vi "PI_GCS2_Sample_Application_With_Analog.vi"() -> ()   [LabVIEW 2020]
doc: "This VI demonstrates the use of digital (e.g. RS-232) communication and analog interfacing in parallel for a PI GCS2 device which can be operated in analog mode. In this example the PI GCS2 device is connected through COM port 1 with baudrate 115200. The VI first initializes the device via the selected digital interface by running PI_GCS2_Configuration_Setup.vi. It then switches to analog control using SwitchToAnalogOrDigital.vi and initializes the analog interface by running Analog_Configuration_Setup.vi. After these initialization steps, it moves one axis relative to its current position by outputting a voltage by the DAC card used, waits 10 ms and queries for the position of this axis. Finally, it switches back to digital control and closes both the analog and the digital connection to the device. \nThe diagram shows how to combine the driver VIs for these tasks. \nWarning: Before running this VI, modify the interface settings to reflect your configuration. The predefined settings provided with the VI probably do not match your system."
uses:
  Low Level/Communication.llb/Interface Settings.ctl
panel:
  out "Running 2":bool caption="Analog_Configuration_Setup.vi is running"
  in  "stop":bool
  in  "error in":errorcluster
  out "Running":bool caption="PI_GCS2_Configuration_Setup.vi is running"
  out "error out":errorcluster
  out "Position":dbl[](array[numeric]) format="%.6f"
  out "Conn. Axis":string[](array[string])
  out "GCS2 Identification":string
  # "This This VI demonstrates the use of digital (e.g. RS-232) communication and analog interfacing in parallel for a PI CGS2 devie that can be operated in analog mode.  The diagram shows how to combine the driver VIs for these tasks.\n\nWarning: Before running this VI, modify the interface settings on the block diagram to reflect your configuration. The predefined \n                 settings provided with the VI probably do not match your system.\n                 Both the PI GCS2 LabVIEW driver set and the GCS Analog LabVIEW driver set must be installed, otherwise the VI will not\n                 be executable."
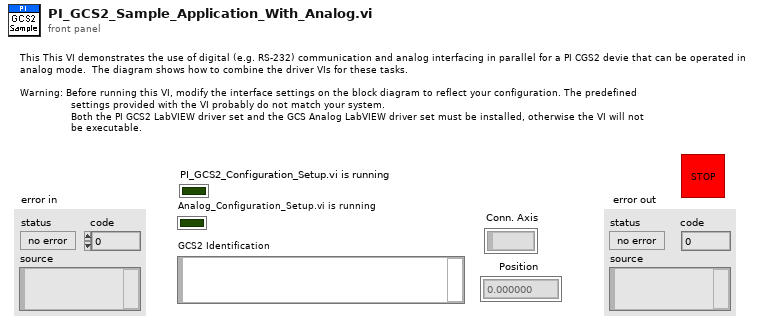
[diagram p1: front panel]
types:
  T1 = typedef "Interface Settings.ctl" = cluster{"Interface":u16, "Timeout":u32, "RS232 settings":cluster{"Portnumber":u8, "Baudrate":u16}, "TCP/IP settings":cluster{"Host address/name":string, "Port":i32, "Board":i32, "TCP/IP Search?":bool}, "USB settings":cluster{"S/N":string, "USB Search?":bool}, "DaisyChain settings":cluster{"Register DC":bool, "DaisyChain Search?":bool, "Device ID":i32}, "DLL for Device":u16}
  T2 = enum16{"Do not reference", "Reference switch", "Negative limit switch", "Positive limit switch"}[]
  T3 = cluster{"Conn. Axes":string[], "AI channels":tag[], "AO channels":tag[], "Lower voltage limit (V)":dbl, "Upper voltage limit (V)":dbl, "AI Sample Rate":dbl, "AI Samples/Channel":i32}
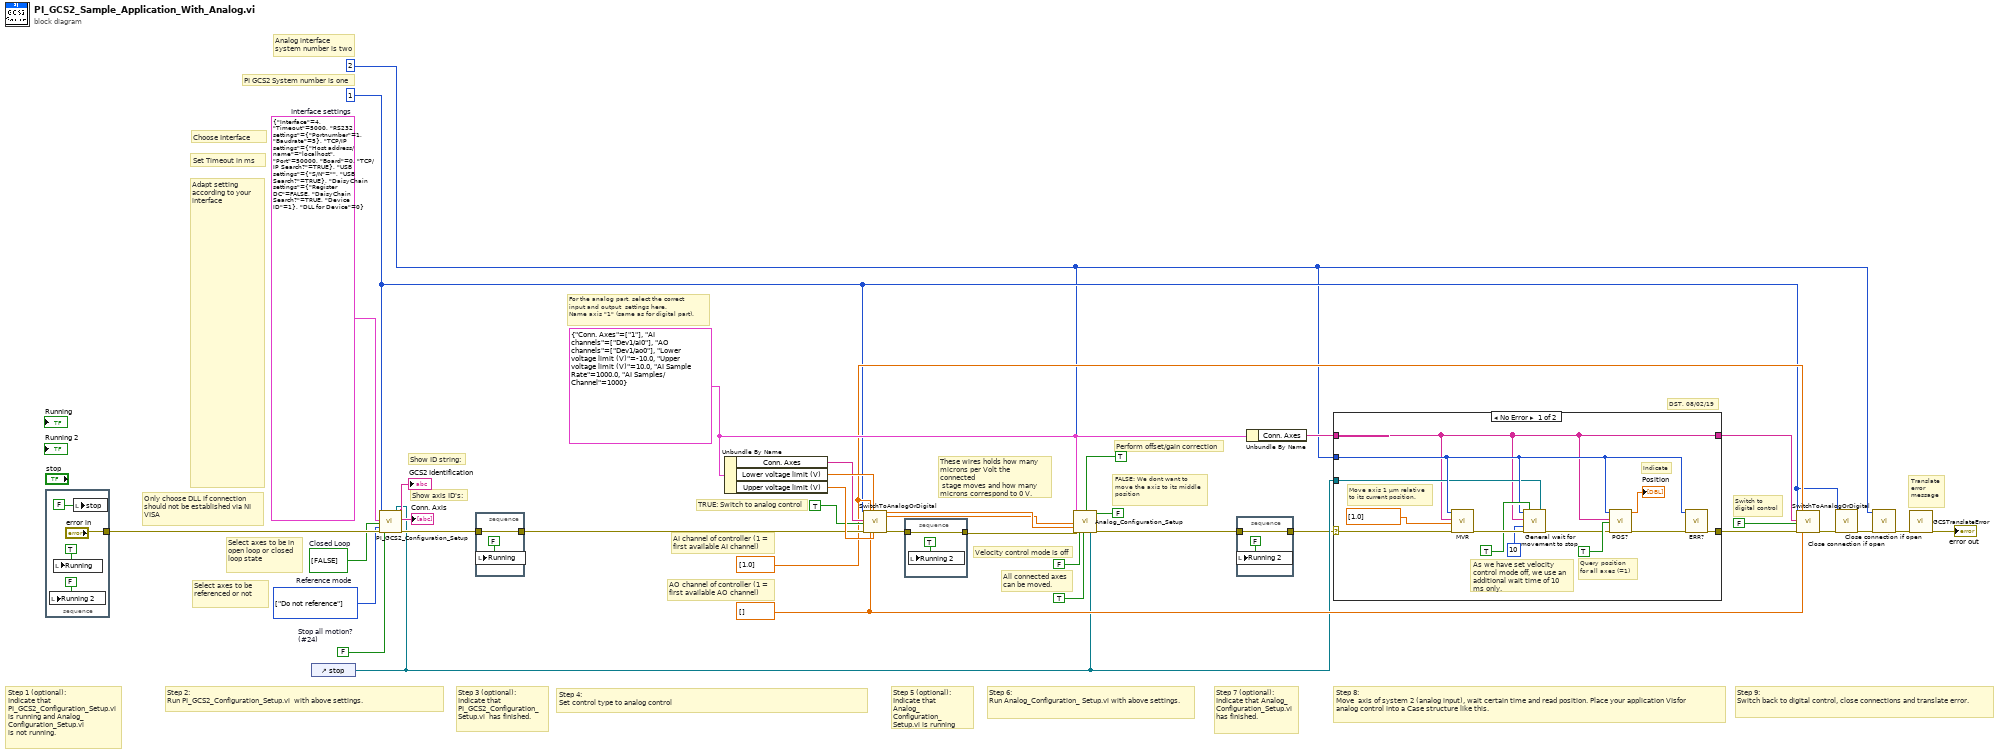
[diagram p0: block diagram]
diagram:
  w6 = T1 {"Interface"=4, "Timeout"=5000, "RS232 settings"={"Portnumber"=1, "Baudrate"=5}, "TCP/IP settings"={"Host address/name"="localhost", "Port"=50000, "Board"=0, "TCP/IP Search?"=TRUE}, "USB settings"={"S/N"="", "USB Search?"=TRUE}, "DaisyChain settings"={"Register DC"=FALSE, "DaisyChain Search?"=TRUE, "Device ID"=1}, "DLL for Device"=0}  # Interface settings
  w8 = FALSE  # Stop all motion? (#24)
  w9 = T2 [enum."Do not reference"] items=["Do not reference", "Reference switch", "Negative limit switch", "Positive limit switch"]  # Reference mode
  w10 = bool[] [FALSE]  # Closed Loop
  w12 = dbl[] [] ("AO channels")
  w13 = dbl[] [1.0] ("AI channels")
  w26 = T3 {"Conn. Axes"=["1"], "AI channels"=["Dev1/ai0"], "AO channels"=["Dev1/ao0"], "Lower voltage limit (V)"=-10.0, "Upper voltage limit (V)"=10.0, "AI Sample Rate"=1000.0, "AI Samples/Channel"=1000} ("Input/output settings")
  w1 = 2 ("System no.")
  w2 = 1 ("System no.")
  # "Select axes to be referenced or not"
  # "Select axes to be in open loop or closed loop state"
  # "Adapt setting according to your interface"
  # "Set Timeout in ms"
  # "Choose Interface"
  # "Only choose DLL if connection should not be established via NI VISA"
  # "DST, 08/02/19"
  # "Step 7 (optional):\nIndicate that Analog_Configuration_Setup.vi has finished."
  # "Step 5 (optional):\nIndicate that\nAnalog_Configuration_\nSetup.vi is running"
  # "Step 3 (optional):\nIndicate that\nPI_GCS2_Configuration_Setup.vi  has finished."
  # "Step 4: \nSet control type to analog control"
  # "Step 9: \nSwitch back to digital control, close connections and translate error."
  # "Translate\nerror \nmessage"
  # "Switch to \ndigital control"
  # "AO channel of controller (1 = \nfirst available AO channel)"
  # "AI channel of controller (1 = \nfirst available AI channel)"
  # "TRUE: Switch to analog control"
  # "Step 6: \nRun Analog_Configuration_ Setup.vi with above settings."
  # "Velocity control mode is off"
  # "FALSE: We dont want to\nmove the axis to its middle\nposition"
  # "Perform offset/gain correction"
  # "All connected axes\ncan be moved."
  # "These wires holds how many\nmicrons per Volt the connected\n stage moves and how many\nmicrons correspond to 0 V."
  # "For the analog part, select the correct \ninput and output  settings here. \nName axis \"1\" (same as for digital part)."
  # "Analog interface \nsystem number is two"
  # "Step 8: \nMove  axis of system 2 (analog input), wait certain time and read position. Place your application VIsfor analog control into a Case structure like this."
  # "Step 2: \nRun PI_GCS2_Configuration_Setup.vi  with above settings."
  # "Step 1 (optional): \nIndicate that\nPI_GCS2_Configuration_Setup.vi\nis running and Analog_\nConfiguration_Setup.vi\nis not running."
  # "Show axis ID's:"
  # "Show ID string:"
  # "PI GCS2 System number is one"
  n1 = stacked-sequence {
    tunnel: ["error in"] -> w11
    frame #0 {
      n2 = local write "Running 2"(FALSE ("Running")) -> ()
      n3 = local write "Running"(TRUE ("Running")) -> ()
      n4 = local write "stop"(FALSE ("stop")) -> ()
    }
  }
  n5 = control-ref of="stop"() -> (w7:refnum<vi>)
  n6 = call "PI_GCS2_Configuration_Setup.vi"("System no."=w2, "Interface settings"=w6, "Closed Loop"=w10, "Reference mode"=w9, "error in"=w11, "Stop all motion?"=w8, "Stop refnum"=w7) -> ("Identification"=→"GCS2 Identification":string, "Conn. Axis"=→"Conn. Axis":string[], "error out"=w18:errorcluster)  [unwired: 6 in, 4 out]
  n7 = stacked-sequence {
    tunnel: w18 -> [w43]
    tunnel: [w43] -> w19
    frame #0 {
      n8 = local write "Running"(FALSE ("Running")) -> ()
    }
  }
  n9 = Unbundle By Name(w26) -> ("Conn. Axes"=w23:string[], "Lower voltage limit (V)"=w31:dbl, "Upper voltage limit (V)"=w30:dbl)
  n10 = call "SwitchToAnalogOrDigital.vi"("System no."=w2, "Axes to command"=w23, "Mode"=TRUE ("Mode (Analog: T)"), "error in"=w19, "AI channels"=w13, "AO channels"=w12, "Lower voltage limit (V)"=w31, "Upper voltage limit (V)"=w30) -> ("Conversion factor"=w28:dbl[], "Offset"=w14:dbl[], "Error out"=w21:errorcluster)  [unwired: 3 in, 6 out]
  n11 = stacked-sequence {
    tunnel: [w44] -> w20
    tunnel: w21 -> [w44]
    frame #0 {
      n12 = local write "Running 2"(TRUE ("Running")) -> ()
    }
  }
  n13 = call "Analog_Configuration_Setup.vi"("System no."=w1, "Input/output settings"=w26, "Conversion offset"=w14, "Conversion factor"=w28, "error in"=w20, "Vel. control mode"=FALSE, "All axes?"=TRUE, "Offset/Gain\ncorrection"=TRUE ("Offset/Gain\ncorrection"), "Move \nto middle?"=FALSE ("Move \nto middle?"), "Stop refnum"=w7) -> ("error out"=w36:errorcluster)  [unwired: 3 in, 6 out]
  n14 = stacked-sequence {
    tunnel: w36 -> [w47]
    tunnel: [w47] -> w5
    frame #0 {
      n15 = local write "Running 2"(FALSE ("Running")) -> ()
    }
  }
  n16 = Unbundle By Name(w26) -> ("Conn. Axes"=w4:string[])
  n17 = case shown="No Error" w5 {
    selector: w5 -> [w49 w62]
    tunnel: [w50 w62] -> w24
    tunnel: w7 -> [w51 _]
    tunnel: w1 -> [w53 _]
    tunnel: w4 -> [w48 w61]
    tunnel: [w48 w61] -> w3
    frame No Error {
      # "As we have set velocity control mode off, we use an additional wait time of 10 ms only."
      # "Indicate"
      # "Query position\nfor all axes (=1)"
      # "Move axis 1 µm relative\nto its current position."
      n18 = call "MVR.vi"("System no."=w53, "Axes to move"=w48, "Position values"=dbl[] [1.0], "error in"=w49) -> ("error out"=w58:errorcluster)  [unwired: 1 in, 14 out]
      n19 = call "General wait for movement to stop.vi"("System no."=w53, "Axes to wait for"=w48, "Additional wait time, ms"=u32 10, "error in"=w58, "Add. wait only?"=TRUE, "Stop refnum"=w51) -> ("error out"=w57:errorcluster)  [unwired: 2 in, 11 out]
      n20 = call "POS?.vi"("System no."=w53, "Axes to query"=w48, "All axes?"=TRUE, "error in"=w57) -> ("Position"=→"Position":dbl[], "error out"=w56:errorcluster)  [unwired: 1 in, 13 out]
      n21 = call "ERR?.vi"("System no."=w53, "error in"=w56) -> ("error out"=w50:errorcluster)  [unwired: 17 out]
    }
    frame Error {
      # "Error during initialization"
    }
  }
  n22 = call "SwitchToAnalogOrDigital.vi"("System no."=w2, "Axes to command"=w3, "Mode"=FALSE, "error in"=w24, "AI channels"=w13, "AO channels"=w12) -> ("Error out"=w17:errorcluster)  [unwired: 3 in, 10 out]
  n23 = call "Close connection if open.vi"("System no."=w2, "error in"=w17) -> ("error out"=w16:errorcluster)  [unwired: 1 in, 16 out]
  n24 = call "Close connection if open.vi"("System no."=w1, "error in"=w16) -> ("error out"=w15:errorcluster)  [unwired: 1 in, 16 out]
  n25 = call "GCSTranslateError.vi"("error in"=w15) -> ("error out"=→"error out":errorcluster)  [unwired: 18 out]
